vi "GSI-HVSwitch2.set channel onOff.vi"(0 "i ref in":refnum<vi>, 1 "on (FALSE)":bool, 2 "channel":i32, 3 "ms timeout (10000)":i32=10000, 5 "error in (no error)":errorcluster) -> (14 "i ref out":refnum<vi>, 17 "timed out":bool, 19 "error out":errorcluster)   [LabVIEW 2014, in "GSI-HVSwitch2.lvlib"]
doc: "Switches the amplifier unit of the device on or off."
uses:
  GSI-HVSwitch2.lvlib
  CSlibraries/UtilityLib/UtilityLib.valueStatus.ctl
  CS_Core/CSApplicationBaseClasses/DeviceBase/DeviceBase.deviceState.ctl
  CS_Core/CSApplicationBaseClasses/PSChannelBase/PSChannelBase.directionType.ctl
  CS_Core/CSApplicationBaseClasses/PSChannelBase/PSChannelBase.serviceType.ctl
  CS_Core/CSApplicationBaseClasses/PSChannelBase/PSChannelBase.statusType.ctl
  CS_Core/CSApplicationBaseClasses/PSChannelBase/PSChannelBase.lvlib
  CSlibraries/UtilityLib/UtilityLib.lvlib
  CS_Core/CSApplicationBaseClasses/DeviceBase/DeviceBase.lvlib
  instr.lib/hvSwitch2/HVSwitch2Driver.lvlib
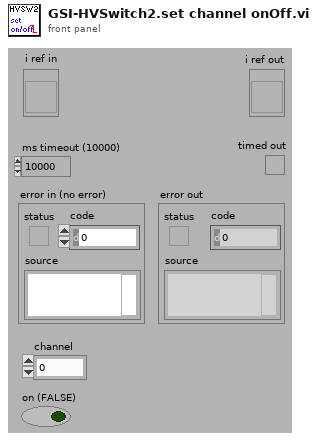
[diagram p1: front panel]
types:
  T1 = typedef "UtilityLib.lvlib/UtilityLib.valueStatus.ctl" = enum16{"no info available", "stand by/off", "on", "warning", "alarm/malfunction", "not implemented", "user action required", "important information", "system default", "control default", "indicator default", "button default"}
  T2 = typedef "PSChannelBase.lvlib/PSChannelBase.serviceType.ctl" = enum16{"onOff", "voltage", "current", "tripCurrent", "rampUpSpeed", "rampDownSpeed", "status"}
  T3 = typedef "GSI-HVSwitch2.lvlib/GSI-HVSwitch2.i attribute.ctl" = cluster{"SDEX VISA Cluster":T4, "SetVoltage SW0":dbl, "SetVoltage SW1":dbl, "ActTempAmp":dbl, "ActTempPS1":dbl, "ActTempPS2":dbl, "mode":T7, "interfaceInitialized":bool, "serviceIDs":cluster{"nomVoltage0ID":i32, "nomVoltage1ID":i32, "actTempAmpID":i32, "actTempPS1ID":i32, "actTempPS2ID":i32, "modeID":i32}, "usedChannels":i32}
  T4 = typedef "SDEXDriver.lvlib/SDEX.VISA Control.ctl" = cluster{"VISA resource name":refnum<visa-resource-name>, "HEX address":u16, "VISA Timeout Value (1000 ms)":u32, "Lock Timeout (1000 ms)":u32, "semaphore":T5, "Baud rate":u32, "revision":T6, "deviceInfo":string}
  T5 = typedef "Semaphore RefNum" = refnum<k1>
  T6 = typedef "SDEXDriver.lvlib/SDEX.revisionType.ctl" = enum16{"unknown", "hvamp3", "hvswi1", "htrp0", "WDG0"}
  T7 = typedef "GSI-HVSwitch2.lvlib/GSI-HVSwitch2.mode.ctl" = enum16{"unknown", "switch", "stepper"}
  T8 = typedef "DeviceBase.lvlib/DeviceBase.deviceState.ctl" = i16
  T9 = typedef "PSChannelBase.lvlib/PSChannelBase.statusType.ctl" = i32
  T10 = typedef "PSChannelBase.lvlib/PSChannelBase.directionType.ctl" = enum16{"unknown", "update actual value", "update nominal value", "update both"}
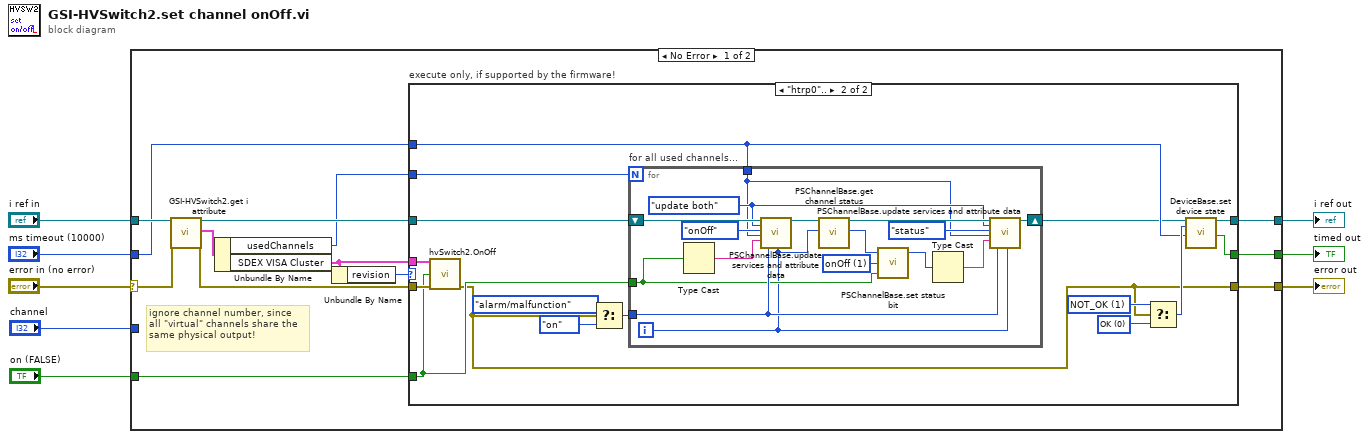
[diagram p0: block diagram]
diagram:
  n1 = case shown="No Error" "error in (no error)" {
    selector: "error in (no error)" -> [w18 w56]
    tunnel: "i ref in" -> [w20 w57]
    tunnel: "ms timeout (10000)" -> [w13 _]
    tunnel: [w12 _] -> w6
    tunnel: [w21 w57] -> w5
    tunnel: [w15 w56] -> w4
    tunnel: "channel" -> [_ _]
    tunnel: "on (FALSE)" -> [w14 _]
    frame No Error {
      # "ignore channel number, since\nall \"virtual\" channels share the\nsame physical output!"
      n2 = call "GSI-HVSwitch2.get i attribute.vi"("i ref in"=w20, "error in (no error)"=w18) -> ("i ref out"=w16:refnum<vi>, "i attribute"=w19:T3, "error out"=w17:errorcluster)  [unwired: 15 in]
      n3 = Unbundle By Name(w19) -> ("usedChannels"=w9:i32, "SDEX VISA Cluster"=w11:T4)
      n4 = Unbundle By Name(w11) -> ("revision"=w10:T6)
      n5 = case "execute only, if supported by the firmware!" shown="\"htrp0\".." w10 {
        tunnel: [w23 w37] -> w21
        tunnel: w17 -> [w22 w33]
        tunnel: w16 -> [w23 w32]
        tunnel: [w22 w24] -> w15
        tunnel: w14 -> [_ w28]
        tunnel: w13 -> [_ w31]
        tunnel: [_ w26] -> w12
        tunnel: w11 -> [_ w29]
        tunnel: w9 -> [_ w25]
        frame Default {
        }
        frame "htrp0".. {
          w35 = T8 1 items=["ERROR"=-1, "OK"=0, "NOT_OK"=1] ("deviceState")
          w36 = T8 0 items=["ERROR"=-1, "OK"=0, "NOT_OK"=1] ("deviceState")
          n6 = call "hvSwitch2.OnOff.vi"("SDEX VISA Cluster"=w29, "on (FALSE)"=w28, "error in (no error)"=w33) -> ("error out"=w24:errorcluster)  [unwired: 11 in, 1 out]
          n7 = Select(t=UtilityLib.valueStatus."alarm/malfunction" ("quality"), s=w24, f=UtilityLib.valueStatus."on") -> (s? t:f=w30:T1)
          n8 = for "for all used channels..." {
            N: w25 -> [_]
            tunnel: w31 -> [w49]
            tunnel: w30 -> [w47]
            tunnel: w28 -> [w44]
            shift-right: [w41] -> w27
            shift-left: w32 -> [w55]
            i -> [w40]
            w45 = T9 1 items=["onOff"=1, "inRange"=2, "rampingUp"=4, "rampingDown"=8, "currentRegulated"=16, "voltageRegulated"=32, "reserved1"=64, "reserved2"=128, "reserved3"=256, "reserved4"=512, "reserved5"=1024, "reserved6"=2048, "reserved7"=4096, "reserved8"=8192, "reserved9"=16384, "reserved10"=32768, "reserved11"=65536, "user1"=131072, "user2"=262144, "user3"=524288, "user4"=1048576, "user5"=2097152, "user6"=4194304, "user7"=8388608, "user8"=16777216, "user9"=33554432, "user10"=67108864, "user11"=134217728, "tripped"=268435456, "warning"=536870912, "error"=1073741824] ("statusBit")
            w51 = PSChannelBase.directionType."update both" ("direction")
            n9 = Type Cast(x=w44) -> (*(type *) &x=w53:string)  [unwired: 1 in]
            n10 = call "PSChannelBase.update services and attribute data.vi"("i ref in"=w55, "direction"=w51, "service"=PSChannelBase.serviceType."onOff", "ms timeout (10000)"=w49, "value"=w53, "quality"=w47, "channelNumber"=w40) -> ("i ref out"=w42:refnum<vi>)  [unwired: 10 in, 2 out]
            n11 = call "PSChannelBase.get channel status.vi"("i ref in"=w42, "channelIndex"=w40) -> ("i ref out"=w52:refnum<vi>, "status"=w46:i32)  [unwired: 15 in, 1 out]
            n12 = call "PSChannelBase.set status bit.vi"("set"=w44, "statusBit"=w45, "status"=w46) -> ("status out"=w43:T9)  [unwired: 2 in]
            n13 = Type Cast(x=w43) -> (*(type *) &x=w48:string)  [unwired: 1 in]
            n14 = call "PSChannelBase.update services and attribute data.vi"("i ref in"=w52, "direction"=w51, "service"=PSChannelBase.serviceType."status", "ms timeout (10000)"=w49, "value"=w48, "quality"=w47, "channelNumber"=w40) -> ("i ref out"=w41:refnum<vi>)  [unwired: 10 in, 2 out]
          }
          n15 = Select(t=w35, s=w24, f=w36) -> (s? t:f=w34:T8)
          n16 = call "DeviceBase.set device state.vi"("i ref in"=w27, "deviceState"=w34, "ms timeout (10000)"=w31) -> ("i ref out"=w37:refnum<vi>, "timed out"=w26:bool)  [unwired: 14 in, 1 out]
        }
      }
    }
    frame Error {
    }
  }
  "error out" <- w4
  "i ref out" <- w5
  "timed out" <- w6
